vi "ReftoDVR.vi"(10 "Ref":u32) -> (2 "DVR":T1)   [LabVIEW 2019, in "RemoteControl.ZMQ.lvlib" / "ZMQ.ContextManager.lvlib"]
uses:
  ZMQ.ContextManager.lvlib
  Context--DVR.ctl
  Context--Cluster.ctl
  <vilib>/addons/zeromq/zmq_context.lvclass
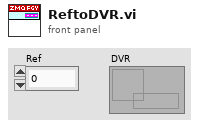
[diagram p1: front panel]
types:
  T1 = typedef "RemoteControl.ZMQ.lvlib/ZMQ.ContextManager.lvlib/Context--DVR.ctl" = refnum<data-value>
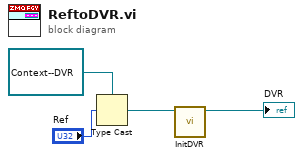
[diagram p0: block diagram]
diagram:
  n1 = Type Cast(type=T1 refnum ("data value reference"), x="Ref") -> (*(type *) &x=w1:T1)
  n2 = call "InitDVR.vi"("DVR"=w1) -> ("DVR"=→"DVR":T1)  [unwired: 9 in, 1 out]
